vi "Update F.vi"(8 "error in (no error)":errorcluster, 10 "SLAM In":T3, 11 "New LM's In":T2(array[cluster])) -> (0 "error out":errorcluster, 2 "SLAM Out":T3, 3 "New LM's Out":T2(array[cluster]))   [LabVIEW 2009]
uses:
  <vilib>/Analysis/Matrix/Datatypes/RealMatrix.ctl
  Controls/SLAM.ctl
  <vilib>/Analysis/Matrix/NI_Matrix.lvlib
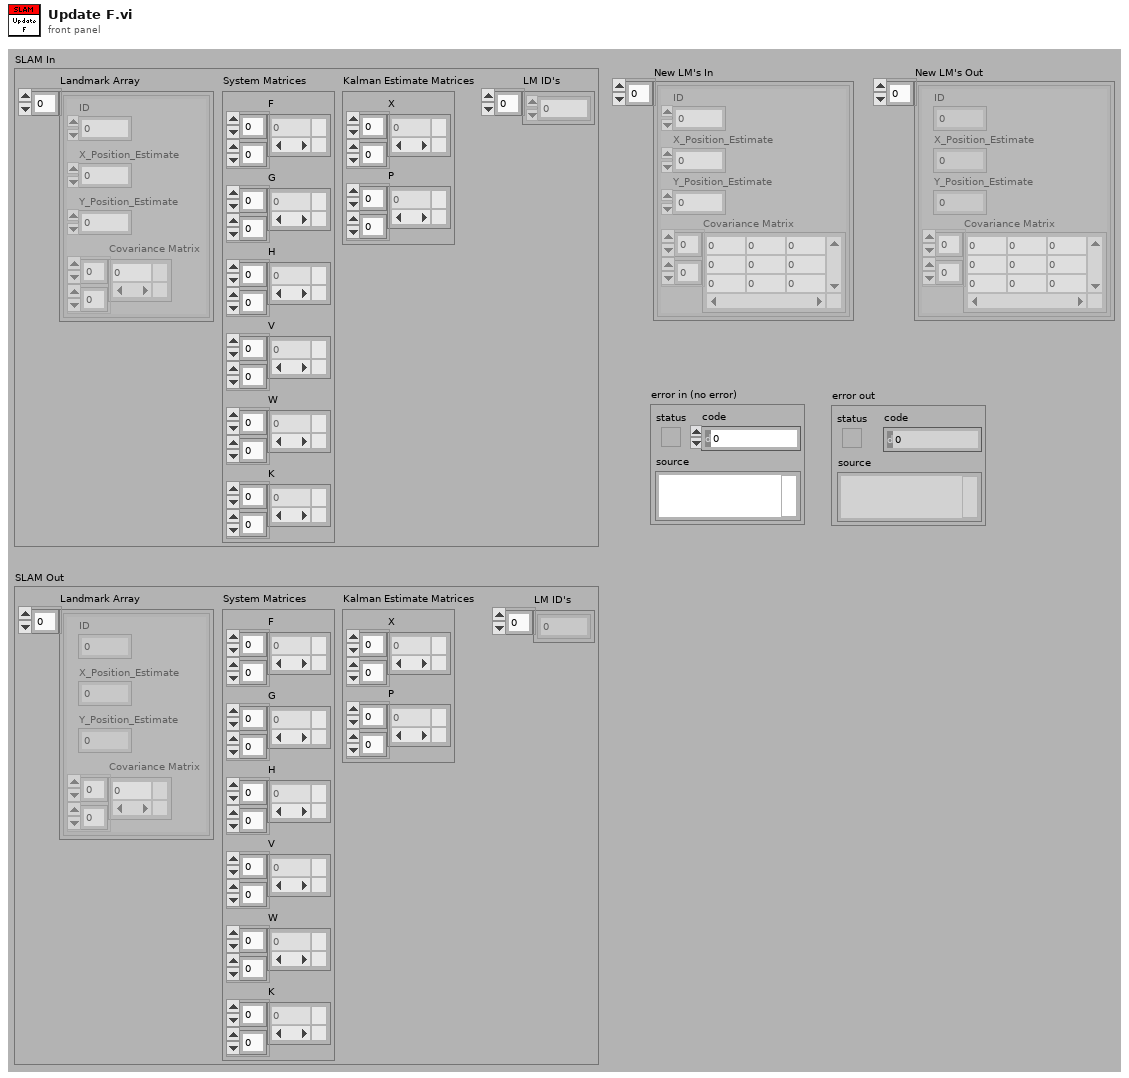
[diagram p1: front panel]
types:
  T1 = typedef "NI_Matrix.lvlib/RealMatrix.ctl" = dbl[][]
  T2 = cluster{"ID":dbl, "X_Position_Estimate":dbl, "Y_Position_Estimate":dbl, "Covariance Matrix":T1}[]
  T3 = typedef "SLAM.ctl" = cluster{"Landmark Array":cluster{"ID":dbl, "X_Position_Estimate":dbl, "Y_Position_Estimate":dbl, "Covariance Matrix":T1}[], "System Matrices":cluster{"F":T1, "G":T1, "H":T1, "V":T1, "W":T1, "K":T1}, "Kalman Estimate Matrices":cluster{"X":T1, "P":T1}, "LM ID's":dbl[]}
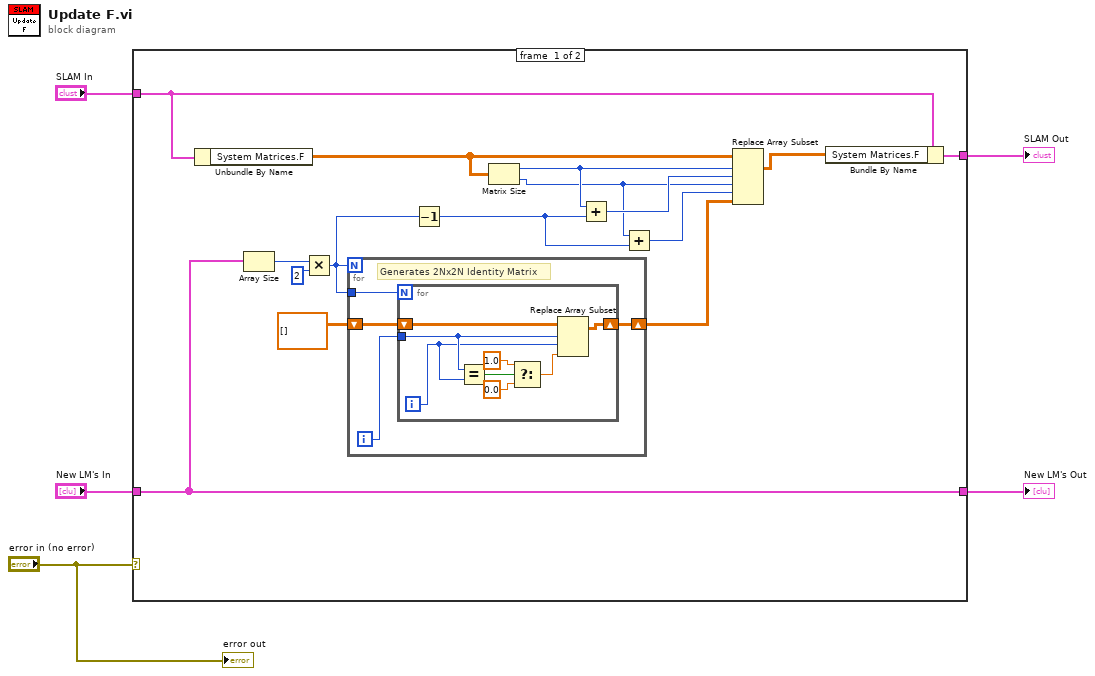
[diagram p0: block diagram]
diagram:
  n1 = case shown="No Error" "error in (no error)" {
    tunnel: "SLAM In" -> [w19 w33]
    tunnel: "New LM's In" -> [w9 w34]
    tunnel: [w12 w33] -> w3
    tunnel: [w9 w34] -> w2
    frame #0 {
      n2 = Unbundle By Name(w19) -> ("System Matrices.F"=w10:T1)
      n3 = Array Size(array=w9) -> (size(s)=w8:i32)
      n4 = Multiply(x=w8, y=2) -> (x*y=w6:i32)
      n5 = for {
        N: w6 -> [_]
        tunnel: w6 -> [w24]
        shift-right: [w21] -> w14
        shift-left: T1 [] ("matrix") -> [w23]
        i -> [w22]
        # "Generates 2Nx2N Identity Matrix"
        n6 = for {
          N: w24 -> [_]
          shift-right: [w31] -> w21
          shift-left: w23 -> [w32]
          tunnel: w22 -> [w30]
          i -> [w29]
          n7 = Equal?(x=w30, y=w29) -> (x = y?=w28:bool)
          n8 = Select(t=1.0 ("new element/submatrix"), s=w28, f=0.0 ("new element/submatrix")) -> (s? t:f=w25:dbl)
          n9 = Replace Array Subset(array=w32, new element=w25, index (row)=w30, index (col)=w29) -> (w31:T1)
        }
      }
      n10 = Decrement(x=w6) -> (x-1=w13:i32)
      n11 = Matrix Size(0:w10) -> (1:w18:i32, 2:w16:i32)
      n12 = Add(x=w18, y=w13) -> (x+y=w17:i32)
      n13 = Add(x=w16, y=w13) -> (x+y=w15:i32)
      n14 = Replace Array Subset(array=w10, new element=w14, index (dim 0)=w18, index (dim 1)=w17, index (dim 2)=w16, index (dim 3)=w15) -> (w11:T1)
      n15 = Bundle By Name(cluster=w19, "System Matrices.F"=w11) -> (w12:T3)
    }
    frame #1 {
    }
  }
  "New LM's Out" <- w2
  "SLAM Out" <- w3
  "error out" <- "error in (no error)"
